vi "Total Images.vi"(8 "error in (no error)":errorcluster, 10 "Total Images":u32, 11 "PLCHandler - Controller -- Interface in":refnum<class "PLCHandler - Controller -- Interface.lvclass">) -> (0 "error out":errorcluster, 3 "PLCHandler - Controller -- Interface out":refnum<class "PLCHandler - Controller -- Interface.lvclass">)   [LabVIEW 2022 SP3, in "PLCHandler - Controller -- Intefrace.lvlib" / "PLCHandler - Controller -- Interface.lvclass"]
uses:
  PLCHandler - Controller -- Interface.lvclass
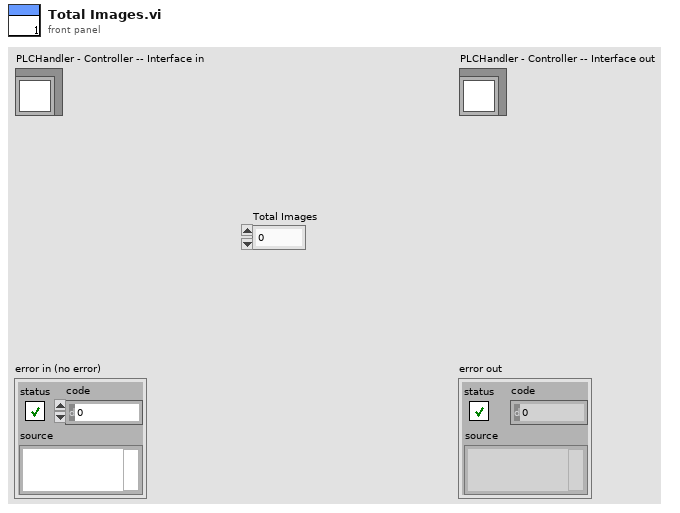
[diagram p1: front panel]
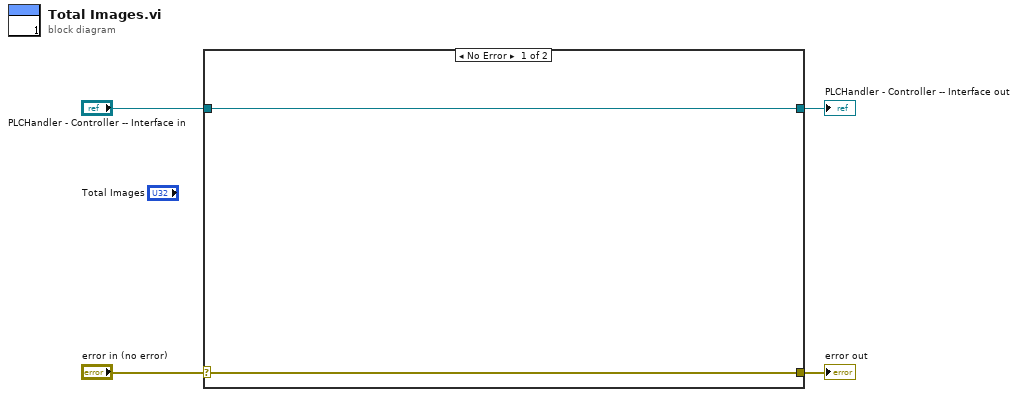
[diagram p0: block diagram]
diagram:
  n1 = case shown="No Error" "error in (no error)" {
    selector: "error in (no error)" -> [w5 w8]
    tunnel: [w5 w8] -> w3
    tunnel: [w6 w7] -> w1
    tunnel: "PLCHandler - Controller -- Interface in" -> [w6 w7]
    frame No Error {
    }
    frame Error {
    }
  }
  "error out" <- w3
  "PLCHandler - Controller -- Interface out" <- w1
